vi "Configure Library on Disk for Development.vi"(10 "save VIs? (T)":bool=TRUE, 11 "library path":path) -> (0 "error out":errorcluster)   [LabVIEW 2020, in "Build Automation.lvlib"]
uses:
  Build Automation.lvlib
panel:
  in  "enable debug? (F)":bool
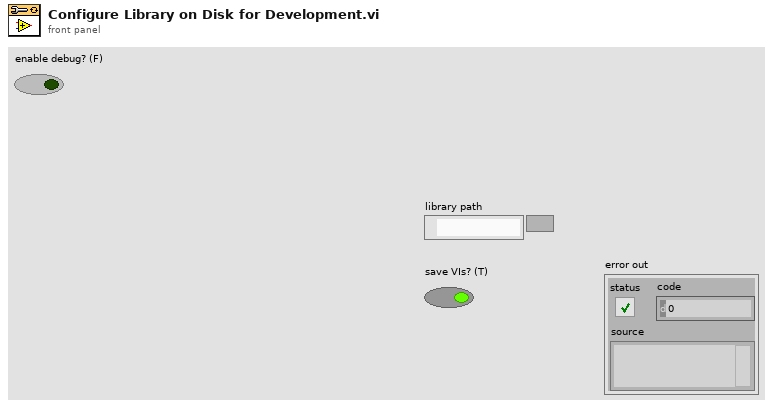
[diagram p1: front panel]
types:
  T1 = enum16{"Share clones between instances", "Preallocate clone for each instance"}
  T2 = cluster{"Status Message":refnum<data-value>, "Progress":refnum<data-value>, "Stop":refnum<data-value>}
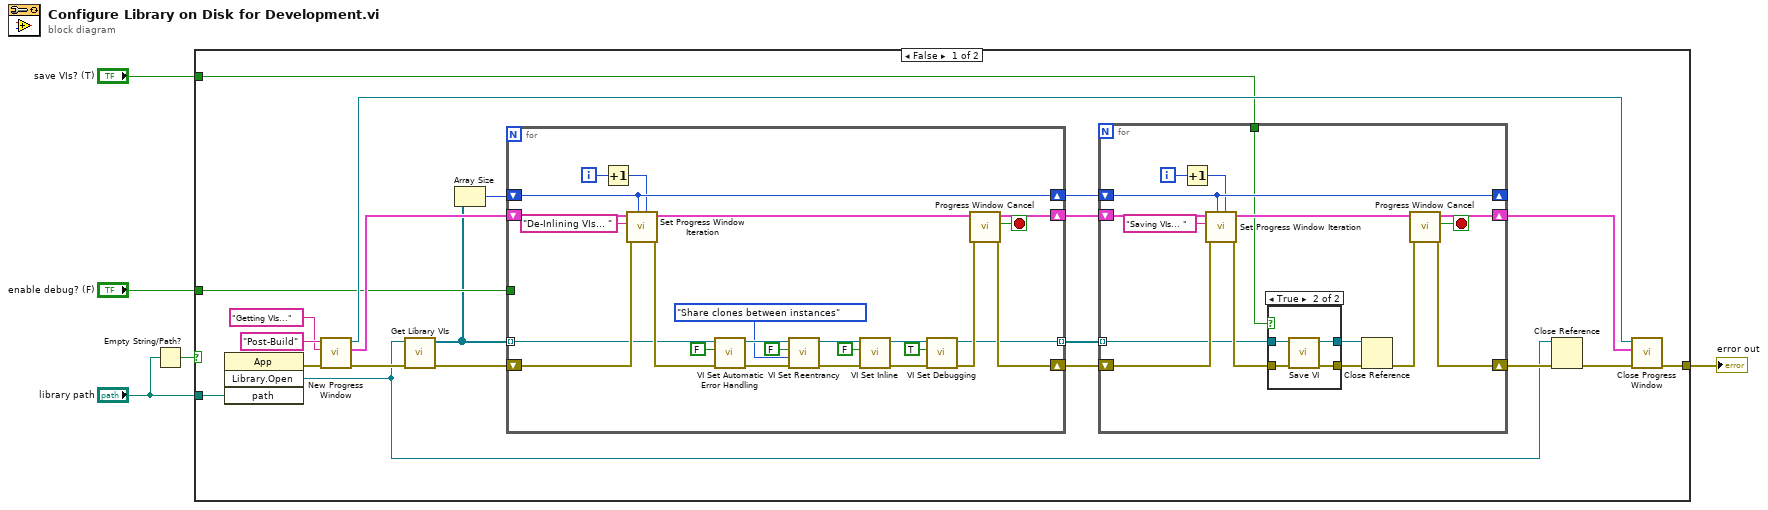
[diagram p0: block diagram]
diagram:
  n1 = Empty String/Path?(string/path="library path") -> (empty?=w4:bool)
  n2 = case shown="False" w4 {
    tunnel: [w21 _] -> w2
    tunnel: "enable debug? (F)" -> [w20 _]
    tunnel: "library path" -> [w12 _]
    tunnel: "save VIs? (T)" -> [w10 _]
    frame False {
      n3 = invoke class="App" method="Library.Open"("path"=w12) -> (error out=w25:errorcluster, "Open Library"=w7:refnum<vi>)  [unwired: 3 in, 2 out]
      n4 = call "New Progress Window.vi"("error in (no error)"=w25, "Initial Message"="Getting VIs...", "Window Title"="Post-Build" ("WindowTitle")) -> ("error out"=w23:errorcluster, "DVRs"=w22:T2, "VI refnum"=w24:refnum<vi>)  [unwired: 6 in]
      n5 = call "Get Library VIs.vi"("error in (no error)"=w23, "library ref"=w7) -> ("error out"=w26:errorcluster, "vi refs"=w18:refnum<vi>[])  [unwired: 8 in]
      n6 = Array Size(array=w18) -> (size(s)=w19:i32)
      n7 = for {
        tunnel: w18 -> [w40] mode=indexing
        shift-right: [w49] -> w16
        shift-left: w22 -> [w45]
        shift-right: [w41] -> w14
        shift-left: w26 -> [w43]
        tunnel: w20 -> [_]
        tunnel: [w29] -> w15 mode=indexing
        shift-right: [w39] -> w17
        shift-left: w19 -> [w39]
        i -> [w51]
        stop <- w50 stop-if-true
        n8 = Increment(x=w51) -> (x+1=w38:i32)
        n9 = call "Set Progress Window Iteration.vi"("current iteration"=w38, "total iterations"=w39, "error in (no error)"=w43, "Status Message"="De-Inlining VIs... ", "DVRs in"=w45) -> ("error out"=w42:errorcluster, "DVRs out"=w44:T2)  [unwired: 5 in]
        n10 = call "VI Set Automatic Error Handling.vi"("error in (no error)"=w42, "Automatic Error Handling"=FALSE, "vi ref in"=w40) -> ("error out"=w46:errorcluster, "vi ref out"=w47:refnum<vi>)  [unwired: 7 in]
        n11 = call "VI Set Reentrancy.vi"("error in (no error)"=w46, "Reentrancy Type (shared clone)"=T1."Share clones between instances", "Is Reentrant"=FALSE, "vi ref in"=w47) -> ("error out"=w33:errorcluster, "vi ref out"=w34:refnum<vi>)  [unwired: 6 in]
        n12 = call "VI Set Inline.vi"("error in (no error)"=w33, "Inline VI"=FALSE, "vi ref in"=w34) -> ("error out"=w31:errorcluster, "vi ref out"=w32:refnum<vi>)  [unwired: 7 in]
        n13 = call "VI Set Debugging.vi"("error in (no error)"=w31, "Allow Debugging"=TRUE, "vi ref in"=w32) -> ("error out"=w30:errorcluster, "vi ref out"=w29:refnum<vi>)  [unwired: 7 in]
        n14 = call "Progress Window Cancel.vi"("error in (no error)"=w30, "DVRs in"=w44) -> ("error out"=w41:errorcluster, "cancelled"=w50:bool, "DVRs out"=w49:T2)  [unwired: 7 in]
      }
      n15 = for {
        tunnel: w15 -> [w53] mode=indexing
        shift-right: [w65] -> w13
        shift-left: w16 -> [w64]
        shift-right: [w61] -> w9
        shift-left: w14 -> [w62]
        shift-right: [w60] -> _
        shift-left: w17 -> [w60]
        tunnel: w10 -> [w52]
        i -> [w67]
        stop <- w66 stop-if-true
        n16 = Increment(x=w67) -> (x+1=w59:i32)
        n17 = call "Set Progress Window Iteration.vi"("current iteration"=w59, "total iterations"=w60, "error in (no error)"=w62, "Status Message"="Saving VIs... ", "DVRs in"=w64) -> ("error out"=w57:errorcluster, "DVRs out"=w63:T2)  [unwired: 5 in]
        n18 = case shown="True" w52 {
          tunnel: w57 -> [w68 w73]
          tunnel: [w69 w72] -> w56
          tunnel: [w68 w71] -> w55
          tunnel: w53 -> [w69 w70]
          frame False {
          }
          frame True {
            n19 = call "Save VI.vi"("error in (no error)"=w73, "vi ref in"=w70) -> ("error out"=w71:errorcluster, "vi ref out"=w72:refnum<vi>)  [unwired: 8 in]
          }
        }
        n20 = Close Reference(reference=w56, error in (no error)=w55) -> (error out=w54:errorcluster)
        n21 = call "Progress Window Cancel.vi"("error in (no error)"=w54, "DVRs in"=w63) -> ("error out"=w61:errorcluster, "cancelled"=w66:bool, "DVRs out"=w65:T2)  [unwired: 7 in]
      }
      n22 = Close Reference(reference=w7, error in (no error)=w9) -> (error out=w8:errorcluster)
      n23 = call "Close Progress Window.vi"("error in (no error)"=w8, "DVRs in"=w13, "VI refnum"=w24) -> ("error out"=w21:errorcluster)  [unwired: 8 in]
    }
    frame True {
    }
  }
  "error out" <- w2
